vi "Wait for Deposit.vi"(8 "entrée d'erreur (pas d'erreur)":errorcluster, 11 "Infos sur le compte":T1) -> (0 "sortie d'erreur":errorcluster, 1 "Arrêter ?":bool, 2 "Montant à créditer":dbl, 3 "Infos sur le compte en sortie":T1)   [LabVIEW 2009]
uses:
  Account Info.ctl
  Stop.vi
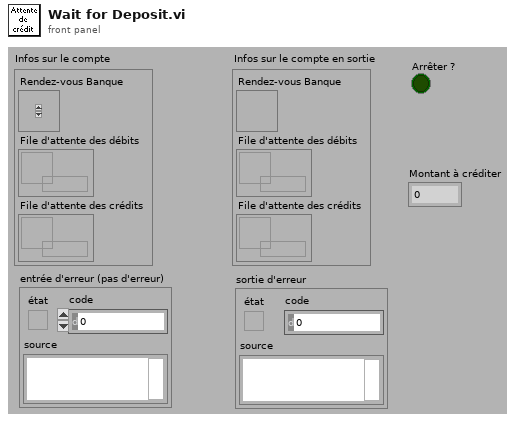
[diagram p1: front panel]
types:
  T1 = typedef "Account Info.ctl" = cluster{"Rendez-vous Banque":T2, "File d'attente des débits":refnum<queue>, "File d'attente des crédits":refnum<queue>}
  T2 = typedef "Rendezvous RefNum" = refnum<k1>
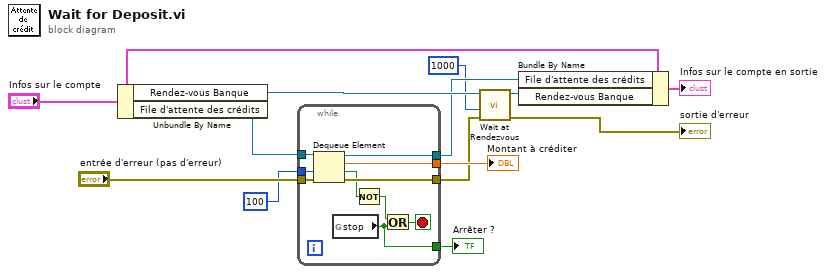
[diagram p0: block diagram]
diagram:
  n1 = Unbundle By Name ("Désassembler par nom")("Infos sur le compte") -> ("Rendez-vous Banque"=w10:T2, "File d'attente des crédits"=w13:refnum<queue>)
  n2 = while "Boucle While" {
    tunnel: w13 -> [w23]
    tunnel: [w22] -> w12
    tunnel: "entrée d'erreur (pas d'erreur)" -> [w21]
    tunnel: [w20] -> w9
    tunnel: [w19] -> w6
    tunnel: 100 ("timeout in ms (-1)") -> [w15]
    tunnel: [w14] -> w1
    stop <- w18 stop-if-true
    n3 = Dequeue Element ("Supprimer le premier élément d'une file d'attente")(queue=w23, timeout in ms (-1)=w15, error in (no error)=w21) -> (queue out=w19:refnum<queue>, element=w22:dbl, timed out?=w16:bool, error out=w20:errorcluster)
    n4 = global read "Stop.vi" "stop"() -> (w14:bool)
    n5 = Not ("Non")(x=w16) -> (.not. x?=w17:bool)
    n6 = Or ("OU")(x=w17, y=w14) -> (x .or. y?=w18:bool)
  }
  "Montant à créditer" <- w12
  "Arrêter ?" <- w1
  n7 = call <vilib>:"Wait at Rendezvous.vi"("error in (no error)"=w9, "ms timeout (-1)"=1000, "rendezvous"=w10) -> ("error out"=→"sortie d'erreur":errorcluster, "rendezvous out"=w7:T2)  [unwired: 3 out]
  n8 = Bundle By Name ("Assembler par nom")(cluster="Infos sur le compte", "File d'attente des crédits"=w6, "Rendez-vous Banque"=w7) -> (→"Infos sur le compte en sortie":T1)
